vi "MM6.InitMCA.vi"(0 "i ref in":refnum<vi>, 2 "InitObjs":string[](array[string]), 3 "ms timeout (10000)":i32=10000, 5 "error in (no error)":errorcluster) -> (14 "i ref out":refnum<vi>, 16 "InitObjs out":string[](array[string]), 17 "timed out":bool, 19 "error out":errorcluster)   [LabVIEW 2014, in "MM6.lvlib"]
doc: "Initializes the MCA (or whatever is taken for data acquisition)"
uses:
  MM6.lvlib
  CSCore/CSSystem/CoreDefs/CoreDefs.call_type.ctl
  CSCore/BaseProcess/BaseProcess.descriptor string definition.ctl
  CSCore/CSSystem/CoreDefs/CoreDefs.rawDataType.ctl
  CSCore/CSSystem/CoreLib/CoreLib.string 2 byte array.vi
  CSCore/CSSystem/CoreLib/CoreLib.int 2 byte array.vi
  CSCore/CSSystem/CoreLib/CoreLib.double 2 byte array.vi
  CSCore/BaseProcess/BaseProcess.lvlib
  LEBITLib/LEBITLib.lvlib
  CSCore/CSSystem/CoreLib/CoreLib.lvlib
panel:
  in  "call cluster type":T1={"Object"="", "Selector"="", "CallType"=enum."synchronous", "Async Object"="", "Async Selector"="", "Data Descriptor"="", "Data"=[], "Error #"=0, "Expire"=0}
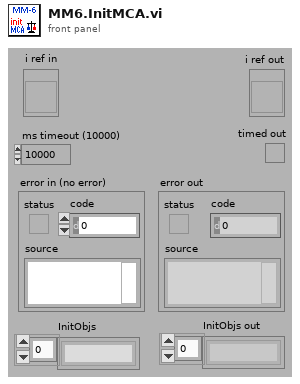
[diagram p1: front panel]
types:
  T1 = typedef "CoreDefs.call_type.ctl" = cluster{"Object":string, "Selector":string, "CallType":enum16{"simple", "synchronous", "asynchronous"}, "Async Object":string, "Async Selector":string, "Data Descriptor":T2, "Data":T3, "Error #":i32, "Expire":u32}
  T2 = typedef "BaseProcess.lvlib/BaseProcess.descriptor string definition.ctl" = string
  T3 = typedef "CoreDefs.rawDataType.ctl" = i8[]
  T4 = typedef "MM6.lvlib/MM6.i attribute.ctl" = cluster{"ConfigData":T5, "UsedObjs":string[], "ActScanStep":i32[], "AbortRequest":bool, "StopRequest":bool, "# cycles":i32, "Connected":bool, "MMStatus":T20, "# data":i32, "DIMServices":cluster{"MM6StatusString":string, "MM6StatusID":i32, "discArchiver":string, "discArchiverID":i32, "eventBuilder":string, "eventBuilderID":i32, "GUIIDString":string, "GUIIDStringID":i32}, "dataFile":string, "ExtraDataSets":T21, "PGRunning":T22}
  T5 = typedef "LEBITDefs.lvlib/LEBITDefs.ConfigData.ctl" = cluster{"GenConfig":T6, "Configs":T8[]}
  T6 = typedef "LEBITDefs.lvlib/LEBITDefs.GenConfig.ctl" = cluster{"Mode":i32, "Logs":T7[]}
  T7 = typedef "LEBITDefs.lvlib/LEBITDefs.Log.ctl" = cluster{"Name":string, "FctName":string, "Special":string}
  T8 = typedef "LEBITDefs.lvlib/LEBITDefs.OneConfig.ctl" = cluster{"MCA":T9, "Timing":T10, "Scans":T13[], "FreqDevs":T14[], "CleanDev":T15, "NrCycles":i32, "Specials":T17[], "Delays":T18[], "DAC":T19}
  T9 = typedef "LEBITDefs.lvlib/LEBITDefs.MCA.ctl" = cluster{"Name":string, "Address":string, "NrChannels":i32, "Gate":i32, "NrPipse":i32}
  T10 = typedef "LEBITDefs.lvlib/LEBITDefs.Timing.ctl" = cluster{"TimeTables":cluster{"TimeTable":T11}[], "Memories":T12[], "ScanX":string, "ScanY":string}
  T11 = typedef "LEBITDefs.lvlib/LEBITDefs.Timetable.ctl" = dbl[]
  T12 = typedef "LEBITDefs.lvlib/LEBITDefs.Memory.ctl" = cluster{"Device":string, "ExtTrig":bool, "TT2Use":i32, "PatternTable":string[]}
  T13 = typedef "LEBITDefs.lvlib/LEBITDefs.ScanDev.ctl" = cluster{"Name":string, "FctName":string, "Values":dbl[], "NrScanVals":i32, "Special":string}
  T14 = typedef "LEBITDefs.lvlib/LEBITDefs.FreqDev.ctl" = cluster{"Name":string, "Amp":dbl, "CenterFreq":dbl, "Time":dbl}
  T15 = typedef "LEBITDefs.lvlib/LEBITDefs.CleanDev.ctl" = cluster{"Name":string, "CleanData":T16[]}
  T16 = typedef "LEBITDefs.lvlib/LEBITDefs.CleanDataType.ctl" = cluster{"Amp":dbl, "Center":dbl, "Plus":dbl, "Minus":dbl, "Time":dbl}
  T17 = typedef "LEBITDefs.lvlib/LEBITDefs.Special.ctl" = cluster{"Name":string, "FctName":string, "VerySpecial":string, "Data":dbl}
  T18 = typedef "LEBITDefs.lvlib/LEBITDefs.Delay.ctl" = cluster{"Name":string, "Delay":dbl}
  T19 = typedef "LEBITDefs.lvlib/LEBITDefs.DAC.ctl" = cluster{"Name":string, "Step1":i32, "Step2":i32}
  T20 = typedef "MM6.lvlib/MM6.status.ctl" = enum16{"loaded", "load_error", "config", "config_error", "init", "init_error", "data_reset", "data_reset_error", "running", "start_error", "run_error", "abort_requested", "aborted", "stop_requested", "stopped", "stop_error", "Connected", "NOTConnected"}
  T21 = typedef "LEBITDefs.lvlib/LEBITDefs.ExtraData.ctl" = cluster{"Ions":cluster{"ExcitIonMass":string, "ExcitIonCharge":i32, "CleanIons":cluster{"CleanIonMass":string, "CleanIonCharge":i32}[]}, "TimingDescription":cluster{"TimeTableDescription":cluster{"Times":string[]}[], "PatternTableDescription":cluster{"Pattern":string[]}[]}, "ScanUnits":string[]}[]
  T22 = typedef "PPG_ABC.lvlib/PPG_ABC.PG_Running.ctl" = i32
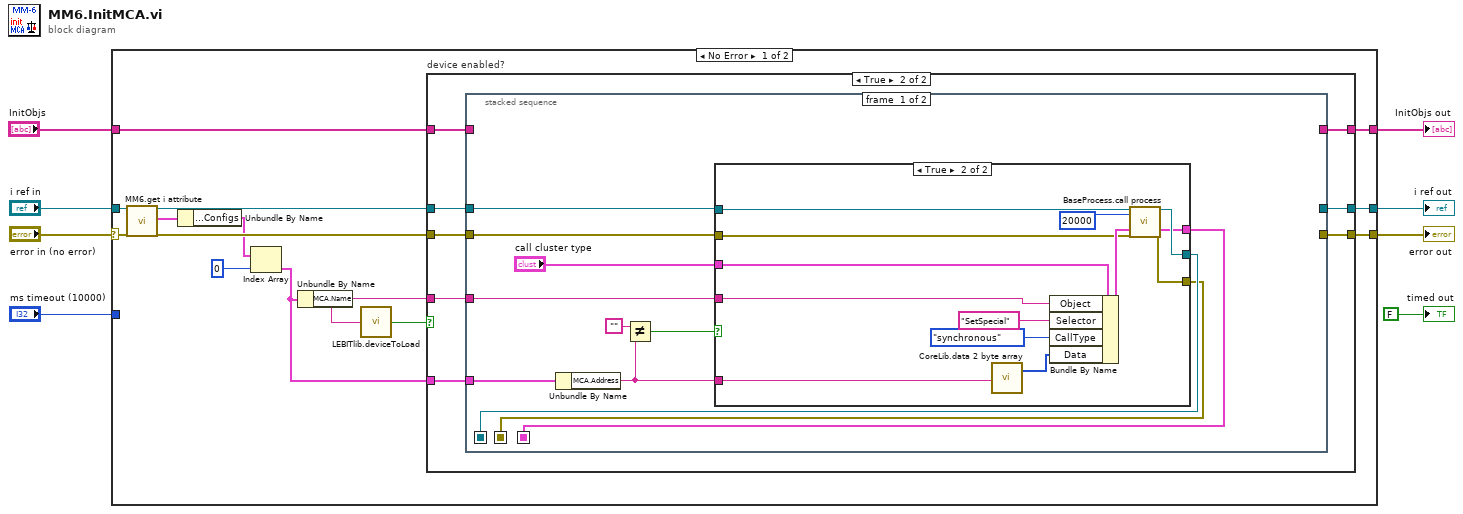
[diagram p0: block diagram]
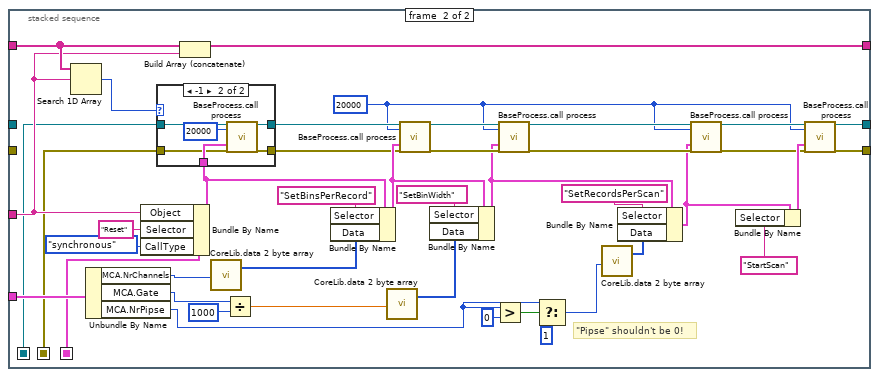
[diagram p4: hidden frame]
diagram:
  n1 = case shown="No Error" "error in (no error)" {
    selector: "error in (no error)" -> [w9 w111]
    tunnel: "i ref in" -> [w22 w113]
    tunnel: [w20 w113] -> w7
    tunnel: [w19 w111] -> w6
    tunnel: "InitObjs" -> [w17 w112]
    tunnel: [w16 w112] -> w3
    tunnel: "ms timeout (10000)" -> [_ _]
    frame No Error {
      n2 = call "MM6.get i attribute.vi"("i ref in"=w22, "error in (no error)"=w9) -> ("i ref out"=w21:refnum<vi>, "i attribute"=w13:T4, "error out"=w18:errorcluster)  [unwired: 15 in]
      n3 = Unbundle By Name(w13) -> ("ConfigData.Configs"=w12:T8[])
      n4 = Index Array(array=w12, index=0) -> (element=w10:T8)
      n5 = Unbundle By Name(w10) -> ("MCA.Name"=w14:string)
      n6 = call "LEBITlib.deviceToLoad.vi"("DeviceName"=w14) -> ("DeviceIsToLoad"=w15:bool)
      n7 = case "device enabled?" shown="True" w15 {
        tunnel: [w25 w33] -> w20
        tunnel: [w24 w32] -> w19
        tunnel: w10 -> [_ w31]
        tunnel: w21 -> [w25 w30]
        tunnel: w18 -> [w24 w29]
        tunnel: w17 -> [w23 w28]
        tunnel: [w23 w27] -> w16
        tunnel: w14 -> [_ w26]
        frame False {
        }
        frame True {
          n8 = stacked-sequence {
            seq-local: [w41 _] -> [_ w75]
            seq-local: [w40 _] -> [_ w74]
            seq-local: [w39 _] -> [_ w73]
            tunnel: [_ w102] -> w33
            tunnel: [_ w101] -> w32
            tunnel: w31 -> [w37 w100]
            tunnel: w30 -> [w42 _]
            tunnel: w29 -> [w44 _]
            tunnel: w28 -> [_ w99]
            tunnel: [_ w98] -> w27
            tunnel: w26 -> [w38 w97]
            frame #0 {
              n9 = Unbundle By Name(w37) -> ("MCA.Address"=w35:string)
              n10 = Not Equal?(x="", y=w35) -> (x != y?=w34:bool)
              n11 = case shown="True" w34 {
                tunnel: w42 -> [w47 w53]
                tunnel: w44 -> [w45 w52]
                tunnel: "call cluster type" -> [w46 w51]
                tunnel: w38 -> [_ w50]
                tunnel: [w47 w57] -> w41
                tunnel: [w45 w56] -> w40
                tunnel: [w46 w55] -> w39
                tunnel: w35 -> [_ w48]
                frame False {
                }
                frame True {
                  n12 = call-poly "CoreLib.data 2 byte array.vi"("string"=w48) -> ("byteArray out"=w49:T3)  [unwired: 18 in]
                  n13 = Bundle By Name(cluster=w51, "Object"=w50, "Selector"="SetSpecial", "CallType"=enum16{"simple", "synchronous", "asynchronous"}."synchronous", "Data"=w49) -> (w58:T1)
                  n14 = call "BaseProcess.call process.vi"("i ref in"=w53, "timeout (ms)"=20000, "call cluster in"=w58, "error in (no error)"=w52) -> ("i ref out"=w57:refnum<vi>, "call cluster out"=w55:T1, "error out"=w56:errorcluster)  [unwired: 13 in]
                }
              }
            }
            frame #1 {
              w61 = 20000 ("timeout (ms)")
              # "\"Pipse\" shouldn't be 0!"
              n15 = Search 1D Array(1D array=w99, element=w97) -> (index of element=w77:i32)  [unwired: 1 in]
              n16 = Unbundle By Name(w100) -> ("MCA.NrChannels"=w63:i32, "MCA.Gate"=w90:i32, "MCA.NrPipse"=w66:i32)
              n17 = Bundle By Name(cluster=w73, "Object"=w97, "Selector"="Reset", "CallType"=enum16{"simple", "synchronous", "asynchronous"}."synchronous") -> (w76:T1)
              n18 = case shown="-1" w77 {
                tunnel: [w104 w109] -> w94
                tunnel: w76 -> [_ w108]
                tunnel: w75 -> [w104 w107]
                tunnel: w74 -> [w103 w106]
                tunnel: [w103 w105] -> w79
                frame 0, Default {
                }
                frame -1 {
                  n19 = call "BaseProcess.call process.vi"("i ref in"=w107, "timeout (ms)"=20000, "call cluster in"=w108, "error in (no error)"=w106) -> ("i ref out"=w109:refnum<vi>, "error out"=w105:errorcluster)  [unwired: 13 in, 1 out]
                }
              }
              n20 = Build Array (concatenate)(w99, w97) -> (w98:string[])
              n21 = call-poly "CoreLib.data 2 byte array.vi"("i32"=w63) -> ("byteArray out"=w71:T3)  [unwired: 18 in]
              n22 = Divide(x=w90, y=1000) -> (x/y=w64:dbl)
              n23 = Bundle By Name(cluster=w76, "Selector"="SetBinsPerRecord", "Data"=w71) -> (w92:T1)
              n24 = call-poly "CoreLib.data 2 byte array.vi"("f64"=w64) -> ("byteArray out"=w72:T3)  [unwired: 18 in]
              n25 = call "BaseProcess.call process.vi"("i ref in"=w94, "timeout (ms)"=w61, "call cluster in"=w92, "error in (no error)"=w79) -> ("i ref out"=w88:refnum<vi>, "error out"=w89:errorcluster)  [unwired: 13 in, 1 out]
              n26 = Bundle By Name(cluster=w92, "Selector"="SetBinWidth", "Data"=w72) -> (w85:T1)
              n27 = Greater?(x=w66, y=0) -> (0:w67:bool)
              n28 = call "BaseProcess.call process.vi"("i ref in"=w88, "timeout (ms)"=w61, "call cluster in"=w85, "error in (no error)"=w89) -> ("i ref out"=w87:refnum<vi>, "error out"=w86:errorcluster)  [unwired: 13 in, 1 out]
              n29 = Select(t=w66, s=w67, f=1) -> (s? t:f=w62:i32)
              n30 = call-poly "CoreLib.data 2 byte array.vi"("i32"=w62) -> ("byteArray out"=w69:T3)  [unwired: 18 in]
              n31 = Bundle By Name(cluster=w85, "Selector"="SetRecordsPerScan", "Data"=w69) -> (w81:T1)
              n32 = call "BaseProcess.call process.vi"("i ref in"=w87, "timeout (ms)"=w61, "call cluster in"=w81, "error in (no error)"=w86) -> ("i ref out"=w83:refnum<vi>, "error out"=w82:errorcluster)  [unwired: 13 in, 1 out]
              n33 = Bundle By Name(cluster=w81, "Selector"="StartScan") -> (w84:T1)
              n34 = call "BaseProcess.call process.vi"("i ref in"=w83, "timeout (ms)"=w61, "call cluster in"=w84, "error in (no error)"=w82) -> ("i ref out"=w102:refnum<vi>, "error out"=w101:errorcluster)  [unwired: 13 in, 1 out]
            }
          }
        }
      }
    }
    frame Error {
    }
  }
  "error out" <- w6
  "i ref out" <- w7
  "InitObjs out" <- w3
  "timed out" <- FALSE ("timed out")
